vi "Read Gobject.vi"(3 "GObject_FPSZ":refnum<class "GObject_FPSZ.lvclass">) -> (1 "GObj Out":refnum<vi>)   [LabVIEW 2016, in "GObject_FPSZ.lvclass"]
uses:
  GObject_FPSZ.lvclass
  GObject_FPSZ.lvclass/GObject_FPSZ.ctl
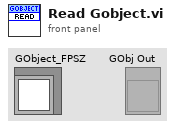
[diagram p1: front panel]
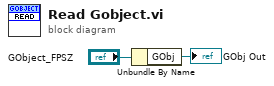
[diagram p0: block diagram]
diagram:
  n1 = Unbundle By Name("GObject_FPSZ") -> ("GObj"=→"GObj Out":refnum<vi>)
